vi "CommGlobal.vi"() -> ()   [LabVIEW 2014]
panel:
  in  "commandmessageType":u32=17476 format="%x"
  in  "commanditems":u8=4
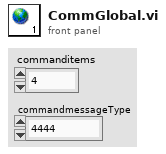
[diagram p1: front panel]
diagram:
